vi "Catch Action Error.vi"(0 "action queue in":refnum<queue>, 1 "TLB' Template in":refnum<class "Synchronize AWS S3 Content TLB`.lvclass">, 11 "error in (no error)":errorcluster, 12 "process state logic enable in":bool) -> (3 "TLB' Template out":refnum<class "Synchronize AWS S3 Content TLB`.lvclass">, 4 "action queue in":refnum<queue>, 14 "process state logic enable out":bool, 15 "error out":errorcluster)   [LabVIEW 2026, in "Synchronize AWS S3 Content.lvlib" / "Synchronize AWS S3 Content TLB`.lvclass"]
uses:
  Synchronize AWS S3 Content TLB`.lvclass
  Actions/System Action Element.ctl
  Application Components/Trigger API/System Trigger.ctl
  Synchronize AWS S3 Content TLB`.lvclass/Synchronize AWS S3 Content TLB`.ctl
  Error Handler/TLB` Error Handler.lvclass/TLB` Error Handler.ctl
  Error Handler/accessors/Set Originating State.vi
  Error Handler/TLB` Error Handler.lvclass
  Actions/Actions.lvlib
  Application Components/Trigger API/Synchronize AWS S3 Content Trigger API.lvlib
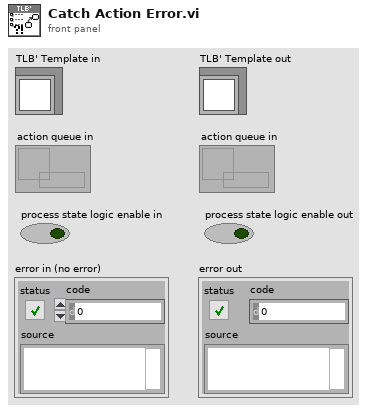
[diagram p1: front panel]
types:
  T1 = typedef "Synchronize AWS S3 Content.lvlib/Synchronize AWS S3 Content Trigger API.lvlib/System Trigger.ctl" = enum16{"<None>", "<Return to Safe State Actions>", "<Cache User Parameters>", "<Close Application>", "<Error>"}
  T2 = typedef "Synchronize AWS S3 Content.lvlib/Synchronize AWS S3 Content TLB`.lvclass/State.ctl" = enum16{"<Startup>", "Idle", "Initiating Configuration", "Validating Commands", "Executing Synchronization", "Validation", "<Shutdown>", "<Error>"}
  T3 = typedef "Synchronize AWS S3 Content.lvlib/Actions.lvlib/System Action Element.ctl" = cluster{"action":string, "data":string}
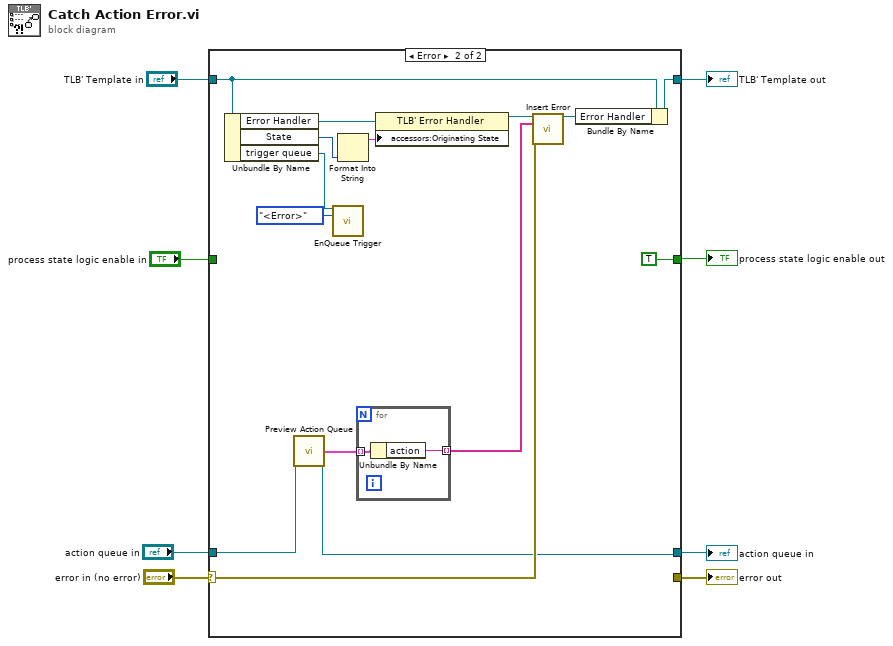
[diagram p0: block diagram]
diagram:
  n1 = case shown="Error" "error in (no error)" {
    selector: "error in (no error)" -> [w12 w26]
    tunnel: [w12 _] -> w3
    tunnel: "TLB' Template in" -> [w10 w23]
    tunnel: "process state logic enable in" -> [w11 _]
    tunnel: [w11 TRUE ("process state logic enable")] -> w6
    tunnel: [w10 w21] -> w8
    tunnel: [w9 w17] -> w1
    tunnel: "action queue in" -> [w9 w19]
    frame No Error {
    }
    frame Error {
      n2 = Unbundle By Name(w23) -> ("Error Handler"=w25:refnum<class "TLB` Error Handler.lvclass">, "State"=w16:T2, "trigger queue"=w14:refnum<queue>)
      n3 = call "Preview Action Queue.vi"("action queue in"=w19) -> ("action queue out"=w17:refnum<queue>, "action elements"=w18:T3[])  [unwired: 12 in, 1 out]
      n4 = call "EnQueue Trigger.vi"("trigger queue in"=w14, "system trigger"=System_Trigger."<Error>") -> ()  [unwired: 12 in, 2 out]
      n5 = Format Into String(w16) -> (resulting string=w15:string)  [unwired: 3 in, 1 out]
      n6 = for {
        tunnel: w18 -> [w29] mode=indexing
        tunnel: [w28] -> w20 mode=indexing
        n7 = Unbundle By Name(w29) -> ("action"=w28:string)
      }
      n8 = property class="TLB' Error Handler"(reference=w25, "accessors:Originating State"=w15) -> (reference out=w24:refnum<class "TLB` Error Handler.lvclass">)  [unwired: 1 in, 1 out]
      n9 = call-dynamic "Insert Error.vi"("error handler in"=w24, "remaining system actions"=w20, "captured error in"=w26) -> ("error handler out"=w22:refnum<class "TLB` Error Handler.lvclass">)  [unwired: 12 in]
      n10 = Bundle By Name(cluster=w23, "Error Handler"=w22) -> (w21:refnum<class "Synchronize AWS S3 Content TLB`.lvclass">)
    }
  }
  "TLB' Template out" <- w8
  "action queue in" <- w1
  "process state logic enable out" <- w6
  "error out" <- w3
